vi "updateLog.vi"(8 "error in (no error)":errorcluster, 10 "model":refnum<class "Model.lvclass">, 11 "AutomatedMotionState in":refnum<class "AutomatedProfileState.lvclass">) -> (0 "error out":errorcluster, 2 "model 2":refnum<class "Model.lvclass">, 3 "AutomatedMotionState out":refnum<class "AutomatedProfileState.lvclass">)   [LabVIEW 2013, in "AutomatedProfileState.lvclass"]
uses:
  AutomatedProfileState.lvclass
  Model/Model/Model.lvclass
  CompensatorActiveState/CompensatorActiveState.lvclass
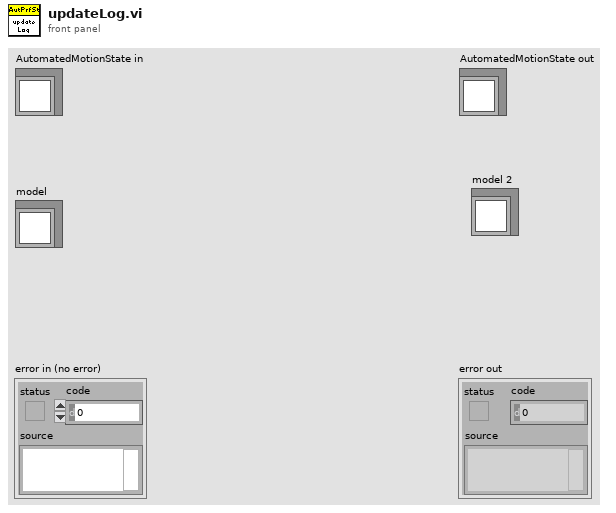
[diagram p1: front panel]
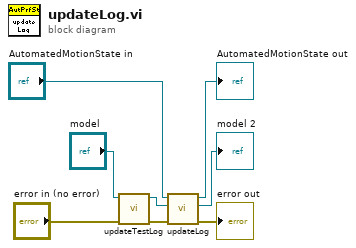
[diagram p0: block diagram]
diagram:
  n1 = call "updateTestLog.vi"("error in (no error)"="error in (no error)", "Model in"="model") -> ("error out"=w1:errorcluster, "Model out"=w3:refnum<class "Model.lvclass">)  [unwired: 8 in]
  n2 = call-parent "updateLog.vi"("error in (no error)"=w1, "model"=w3, "State in"="AutomatedMotionState in") -> ("error out"=→"error out":errorcluster, "model 2"=→"model 2":refnum<class "Model.lvclass">, "State out"=→"AutomatedMotionState out":refnum<class "AutomatedProfileState.lvclass">)  [unwired: 6 in]
